vi "XY plotter leader program.vi"() -> ()   [LabVIEW 2019]
uses:
  SubVi/Dummy.ctl
  <vilib>/Utility/file.llb/Write Delimited Spreadsheet (string).vi
  <vilib>/Utility/file.llb/Write Delimited Spreadsheet (DBL).vi
panel:
  out "new file path (Not A Path if cancelled)":path caption="Path for the saved result"
  out "Array":dbl[](array[numeric]) caption="Measured Result"
  out "Enum":T1 caption="Current Procedure"
  out "Numeric_ Control":i32 caption="Number of coordinate"
  out "OutputValues":dbl[](array[numeric]) caption="Final OutputValues"
  in  "Input":dbl[][](array[numeric])=[[12.0, 10.0], [12.0, 26.0], [12.0, 42.0], [12.0, 58.0], [12.0, 74.0], [12.0, 90.0], [31.0, 10.0], [31.0, 26.0], [31.0, 42.0], [31.0, 58.0], [31.0, 74.0], [31.0, 90.0], [50.0, 10.0], [50.0, 26.0], [50.0, 42.0], [50.0, 58.0], [50.0, 74.0], [50.0, 90.0], [69.0, 10.0], [69.0, 26.0], [69.0, 42.0], [69.0, 58.0], [69.0, 74.0], [69.0, 90.0], [88.0, 10.0], [88.0, 26.0], [88.0, 42.0], [88.0, 58.0], [88.0, 74.0], [88.0, 90.0]] caption="Input Coordinate"
  in  "Stop Button":bool
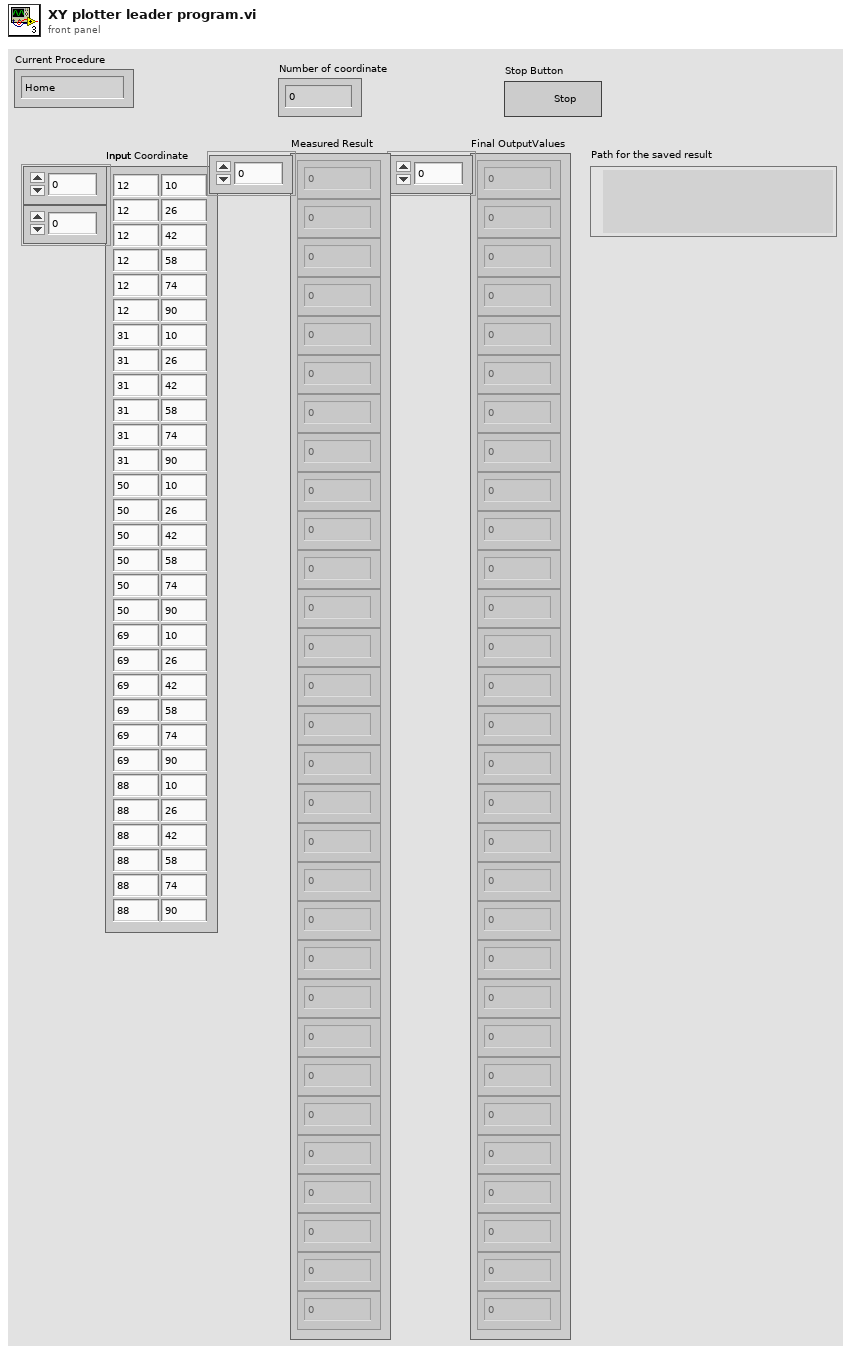
[diagram p1: front panel]
types:
  T1 = typedef "Dummy.ctl" = enum16{"Home", "SendCoords", "Send Measure", "ReadMeasurement", "End"}
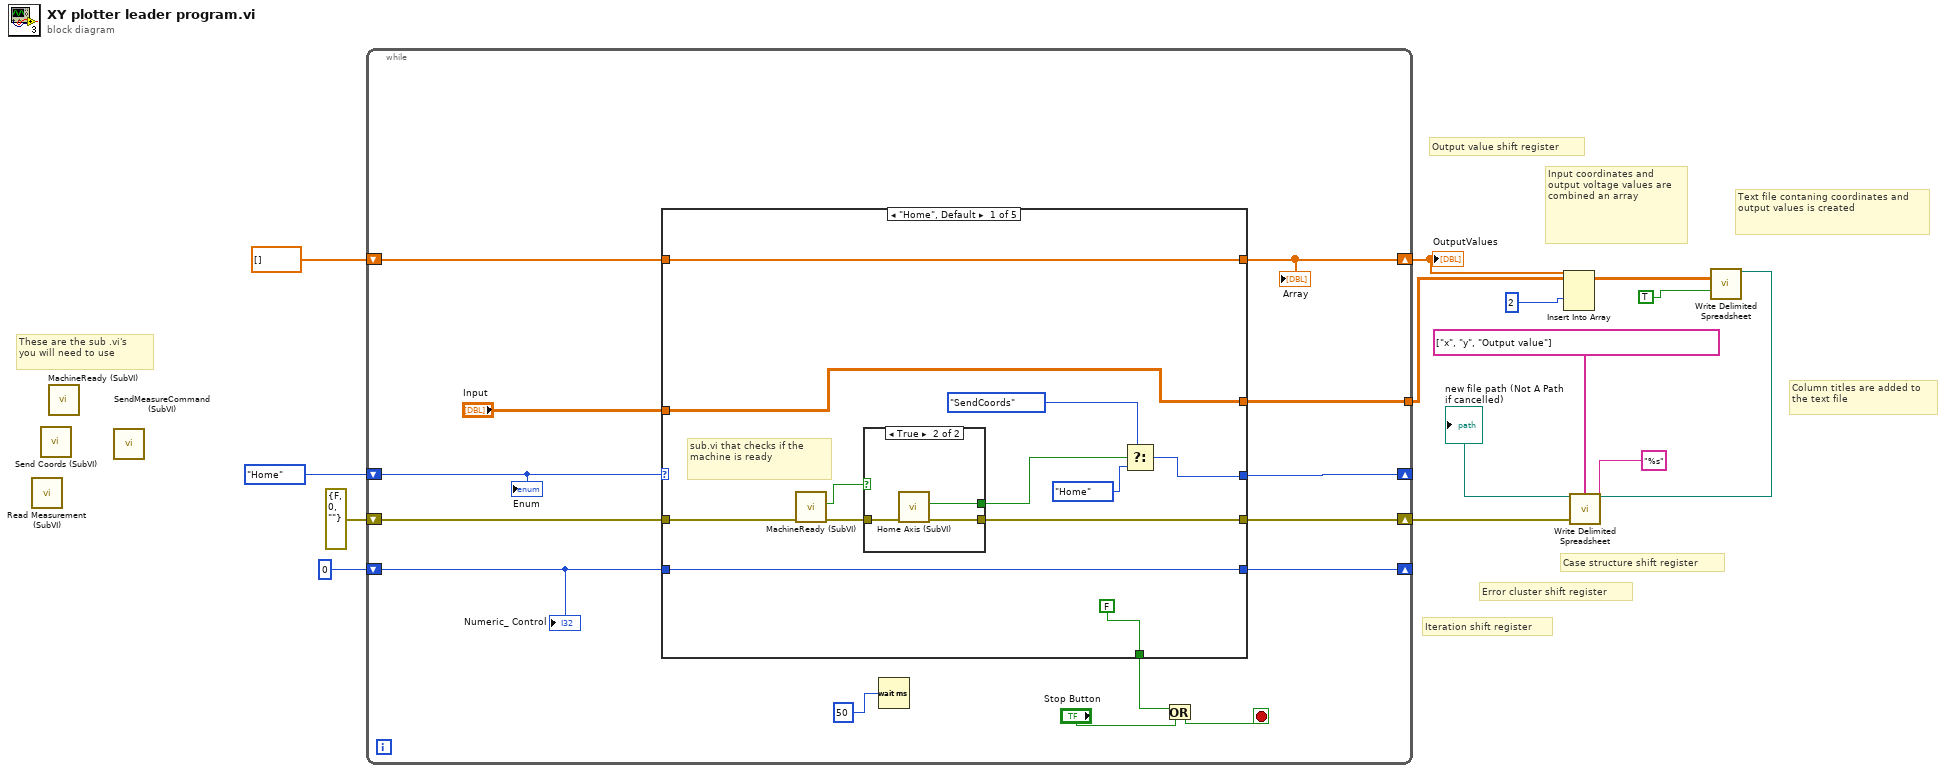
[diagram p0: block diagram]
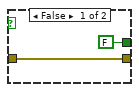
[diagram p2: hidden frame]
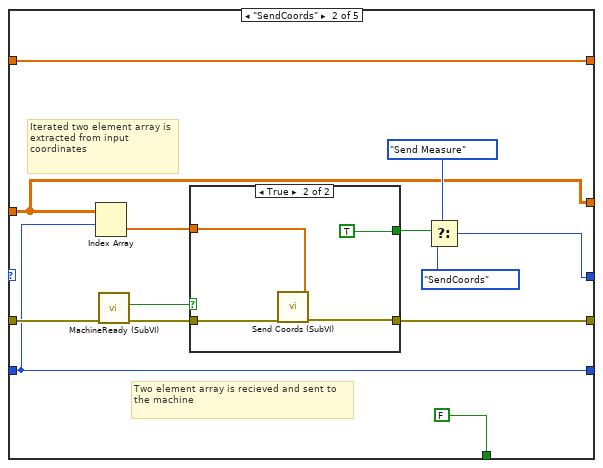
[diagram p3: hidden frame]
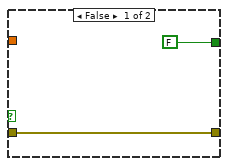
[diagram p4: hidden frame]
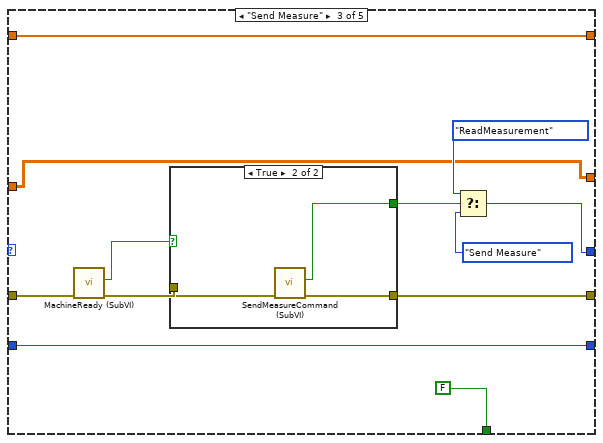
[diagram p5: hidden frame]
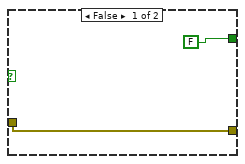
[diagram p6: hidden frame]
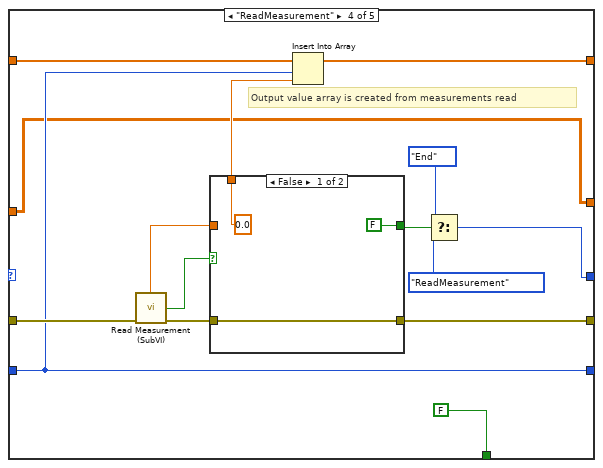
[diagram p7: hidden frame]
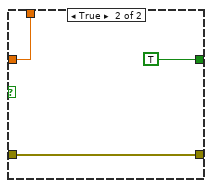
[diagram p8: hidden frame]
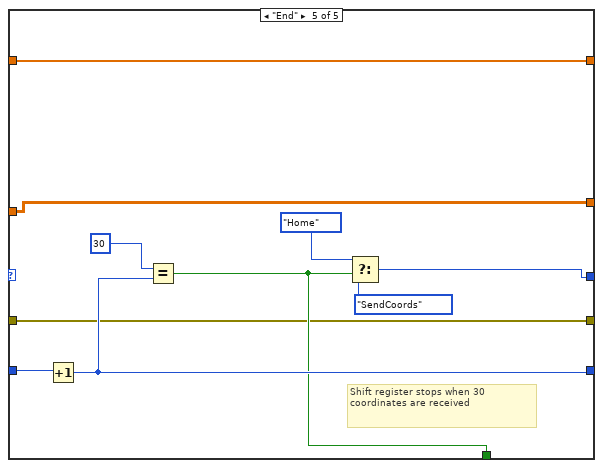
[diagram p9: hidden frame]
diagram:
  # "Output value shift register"
  # "Case structure shift register"
  # "Error cluster shift register"
  # "Iteration shift register"
  # "Text file contaning coordinates and output values is created"
  # "Column titles are added to the text file"
  # "Input coordinates and output voltage values are combined an array"
  # "These are the sub .vi's \nyou will need to use"
  n1 = call "Read Measurement (SubVI).vi"() -> ()  [unwired: 9 in, 3 out]
  n2 = call "Send Coords (SubVI).vi"() -> ()  [unwired: 11 in, 1 out]
  n3 = call "MachineReady (SubVI).vi"() -> ()  [unwired: 10 in, 2 out]
  n4 = call "SendMeasureCommand (SubVI).vi"() -> ()  [unwired: 10 in, 2 out]
  n5 = while {
    shift-right: [w25] -> _
    shift-left: Dummy."Home" -> [w20]
    shift-right: [w14] -> _
    shift-left: 0 -> [w24]
    shift-right: [w21] -> w7
    shift-left: errorcluster {"status"=FALSE, "code"=0, "source"=""} ("error constant") -> [w22]
    shift-right: [w18] -> w8
    shift-left: dbl[] [] -> [w19]
    tunnel: [w15] -> w9
    stop <- w17 stop-if-true
    n6 = case shown="\"Home\", Default" w20 {
      tunnel: [w37 w49 w66 w84 w104] -> w25
      tunnel: w24 -> [w35 w46 w69 w93 w110]
      tunnel: [w35 w46 w69 w93 w109] -> w14
      tunnel: "Input" -> [w28 w45 w64 w81 w102]
      tunnel: w22 -> [w32 w57 w73 w95 w103]
      tunnel: [w30 w55 w75 w83 w103] -> w21
      tunnel: w19 -> [w34 w47 w70 w94 w111]
      tunnel: [w34 w47 w70 w92 w111] -> w18
      tunnel: [FALSE FALSE FALSE FALSE w107] -> w16
      tunnel: [w28 w45 w64 w81 w102] -> w15
      frame "Home", Default {
        # "sub.vi that checks if the machine is ready"
        n7 = call "MachineReady (SubVI).vi"("Error In"=w32) -> ("Error Out"=w31:errorcluster, "Ready?"=w29:bool)  [unwired: 9 in]
        n8 = case shown="True" w29 {
          tunnel: [FALSE ("Sent Command?") w44] -> w36
          tunnel: w31 -> [w40 w43]
          tunnel: [w40 w42] -> w30
          frame False {
          }
          frame True {
            n9 = call "Home Axis (SubVI).vi"("Error In"=w43) -> ("Error Out"=w42:errorcluster, "Sent Command?"=w44:bool)  [unwired: 7 in]
          }
        }
        n10 = Select(t=Dummy."SendCoords", s=w36, f=Dummy."Home") -> (s? t:f=w37:T1)
      }
      frame "SendCoords" {
        # "Two element array is recieved and sent to the machine"
        # "Iterated two element array is extracted from input coordinates"
        n11 = Index Array(array=w45, index (row)=w46) -> (element=w53:dbl[])  [unwired: 1 in]
        n12 = call "MachineReady (SubVI).vi"("Error In"=w57) -> ("Error Out"=w54:errorcluster, "Ready?"=w56:bool)  [unwired: 9 in]
        n13 = case shown="True" w56 {
          tunnel: [w59 w61] -> w55
          tunnel: w54 -> [w59 w62]
          tunnel: w53 -> [_ w63]
          tunnel: [FALSE TRUE] -> w51
          frame False {
          }
          frame True {
            n14 = call "Send Coords (SubVI).vi"("Error In"=w62, "Coordinates"=w63) -> ("Error Out"=w61:errorcluster)  [unwired: 9 in]
          }
        }
        n15 = Select(t=Dummy."Send Measure" ("Enum"), s=w51, f=Dummy."SendCoords" ("Enum")) -> (s? t:f=w49:T1)
      }
      frame "Send Measure" {
        n16 = call "MachineReady (SubVI).vi"("Error In"=w73) -> ("Error Out"=w72:errorcluster, "Ready?"=w71:bool)  [unwired: 9 in]
        n17 = case shown="True" w71 {
          tunnel: w72 -> [w76 w80]
          tunnel: [w76 w79] -> w75
          tunnel: [FALSE w78] -> w74
          frame False {
          }
          frame True {
            n18 = call "SendMeasureCommand (SubVI).vi"("error in (no error)"=w80) -> ("error out"=w79:errorcluster, "Command Sent?"=w78:bool)  [unwired: 9 in]
          }
        }
        n19 = Select(t=Dummy."ReadMeasurement" ("Enum"), s=w74, f=Dummy."Send Measure" ("Enum")) -> (s? t:f=w66:T1)
      }
      frame "ReadMeasurement" {
        # "Output value array is created from measurements read"
        n20 = call "Read Measurement (SubVI).vi"("Error In"=w95) -> ("Error Out"=w91:errorcluster, "Measurement recieved?"=w90:bool, "Measurement Out"=w88:dbl)  [unwired: 8 in]
        n21 = case shown="False" w90 {
          tunnel: [w98 w101] -> w83
          tunnel: w91 -> [w98 w101]
          tunnel: [0.0 w100] -> w89
          tunnel: w88 -> [_ w100]
          tunnel: [FALSE TRUE] -> w85
          frame False {
          }
          frame True {
          }
        }
        n22 = Insert Into Array(array=w94, index=w93, new element=w89) -> (w92:dbl[])
        n23 = Select(t=Dummy."End" ("Enum"), s=w85, f=Dummy."ReadMeasurement" ("Enum")) -> (s? t:f=w84:T1)
      }
      frame "End" {
        # "Shift register stops when 30 coordinates are received"
        n24 = Increment(x=w110) -> (x+1=w109:i32)
        n25 = Equal?(x=30, y=w109) -> (x = y?=w107:bool)
        n26 = Select(t=Dummy."Home" ("Enum"), s=w107, f=Dummy."SendCoords" ("Enum")) -> (s? t:f=w104:T1)
      }
    }
    "Array" <- w18
    n27 = Wait (ms)(milliseconds to wait=u16 50) -> ()  [unwired: 1 out]
    n28 = Or(x=w16, y="Stop Button") -> (x .or. y?=w17:bool)
    "Numeric_ Control" <- w24
    "Enum" <- w20
  }
  "OutputValues" <- w8
  n29 = Insert Into Array(array=w9, index (col)=2, new element=w8) -> (w2:dbl[][])  [unwired: 1 in]
  n30 = call-poly <vilib>:"Write Delimited Spreadsheet.vi"("format (%s)"="%s", "1D data"=string[] ["x", "y", "Output value"], "error in (no error)"=w7) -> ("new file path (Not A Path if cancelled)"=w1:path)  [unwired: 11 in, 1 out]
  "new file path (Not A Path if cancelled)" <- w1
  n31 = call-poly <vilib>:"Write Delimited Spreadsheet.vi"("file path (dialog if empty)"=w1, "2D data"=w2, "append to file? (new file:F)"=TRUE) -> ()  [unwired: 11 in, 2 out]
